vi "dfd_Group Delay_Line Search.vi"(6 "Gradient":cluster{"r":dbl[], "theta":dbl[], "tau":dbl}, 7 "steplength (in)":dbl, 9 "error (in)":dbl, 10 "Coefficients (in)":cluster{"r":dbl[], "theta":dbl[], "offset":dbl}, 11 "Design Info":T1={"p"=2, "freq grid"=[], "d"=[], "weight"=[], "Order"=0, "radius"=1.0}) -> (1 "error (out)":dbl, 2 "Coefficients (out)":cluster{"r":dbl[], "theta":dbl[], "offset":dbl}, 3 "Design Info (dup)":T1={"p"=2, "freq grid"=[], "d"=[], "weight"=[], "Order"=0, "radius"=1.0}, 4 "success":bool, 5 "steplength (out)":dbl)   [LabVIEW 2017, in "NI_DigFilter_Design.lvlib"]
uses:
  <vilib>/addons/Digital Filter Design/NI_DigFilter_Design.lvlib
  <vilib>/addons/Digital Filter Design/_GroupDelay.llb/dfd_Group Delay_Design Info.ctl
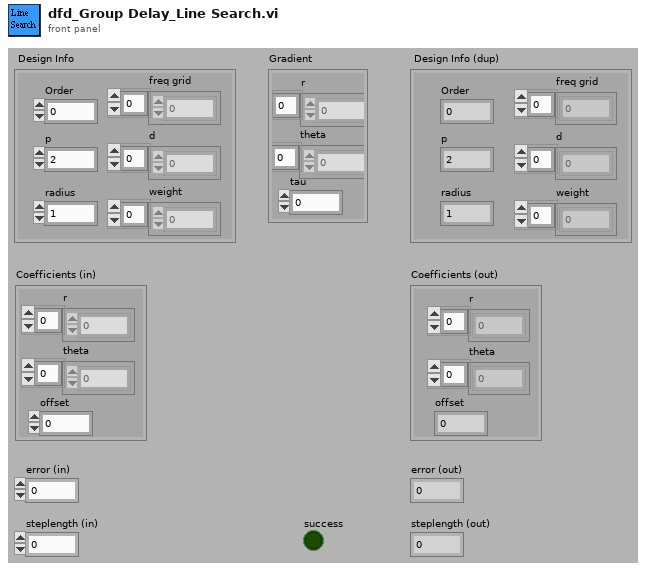
[diagram p1: front panel]
types:
  T1 = typedef "dfd_Group Delay_Design Info.ctl" = cluster{"p":i32, "freq grid":dbl[], "d":dbl[], "weight":dbl[], "Order":i32, "radius":dbl}
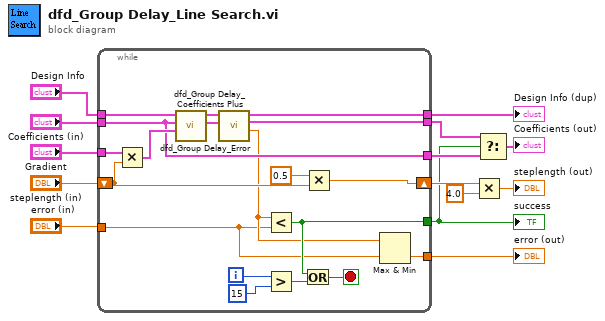
[diagram p0: block diagram]
diagram:
  n1 = while {
    tunnel: "Coefficients (in)" -> [w19]
    tunnel: "Design Info" -> [w25]
    tunnel: "error (in)" -> [w16]
    shift-right: [w29] -> w10
    shift-left: "steplength (in)" -> [w23]
    tunnel: "Gradient" -> [w33]
    tunnel: [w18] -> w6
    tunnel: [w19] -> w7
    tunnel: [w20] -> w8
    tunnel: [w21] -> w9
    tunnel: [w15] -> w5
    i -> [w32]
    stop <- w27 stop-if-true
    n2 = Multiply(x=w33, y=w23) -> (x*y=w24:cluster{"r":dbl[], "theta":dbl[], "tau":dbl})
    n3 = call <vilib>:"dfd_Group Delay_Coefficients Plus.vi"("Gradients"=w24, "Coefficients (in)"=w19, "Group Delay Design Info"=w25) -> ("Coefficients (out)"=w26:cluster{"r":dbl[], "theta":dbl[], "offset":dbl}, "Group Delay Design Info (dup)"=w22:T1)  [unwired: 1 in, 6 out]
    n4 = call <vilib>:"dfd_Group Delay_Error.vi"("Coefficients"=w26, "Design Info"=w22) -> ("Error"=w17:dbl, "Coefficients (dup)"=w20:cluster{"r":dbl[], "theta":dbl[], "offset":dbl}, "Design Info (dup)"=w21:T1)  [unwired: 1 in, 6 out]
    n5 = Less?(x=w17, y=w16) -> (x < y?=w18:bool)
    n6 = Greater?(x=w32, y=15) -> (0:w30:bool)
    n7 = Or(x=w18, y=w30) -> (x .or. y?=w27:bool)
    n8 = Multiply(x=0.5, y=w23) -> (x*y=w29:dbl)
    n9 = Max & Min(x=w17, y=w16) -> (min(x,y)=w15:dbl)  [unwired: 1 out]
  }
  "Design Info (dup)" <- w9
  "success" <- w6
  "error (out)" <- w5
  n10 = Multiply(x=w10, y=4.0) -> (x*y=→"steplength (out)":dbl)
  n11 = Select(t=w8, s=w6, f=w7) -> (s? t:f=→"Coefficients (out)":cluster{"r":dbl[], "theta":dbl[], "offset":dbl})
